vi "LuaVIEW Parse Library Infos.vi"(7 "library path":path, 11 "error in (no error)":errorcluster) -> (8 "library infos":T1[](array[typedef]), 15 "error out":errorcluster)   [LabVIEW 2012]
doc: "Extracts docstrings from a function library and builds a list of function infos."
uses:
  typedefs/clusters/LuaVIEW Function Info.ctl
  served/LuaVIEW Check Synopsis_srv.ctl
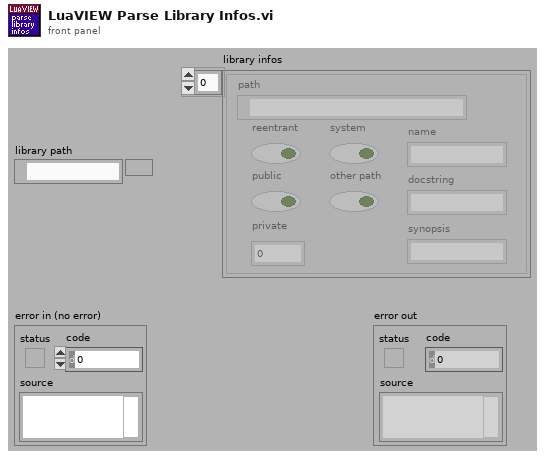
[diagram p1: front panel]
types:
  T1 = typedef "LuaVIEW Function Info.ctl" = cluster{"path":path, "reentrant":bool, "public":bool, "private":i32, "system":bool, "other path":bool, "name":string, "docstring":string, "synopsis":string}
  T2 = typedef "LuaVIEW Check Synopsis_srv.ctl" = refnum<vi>
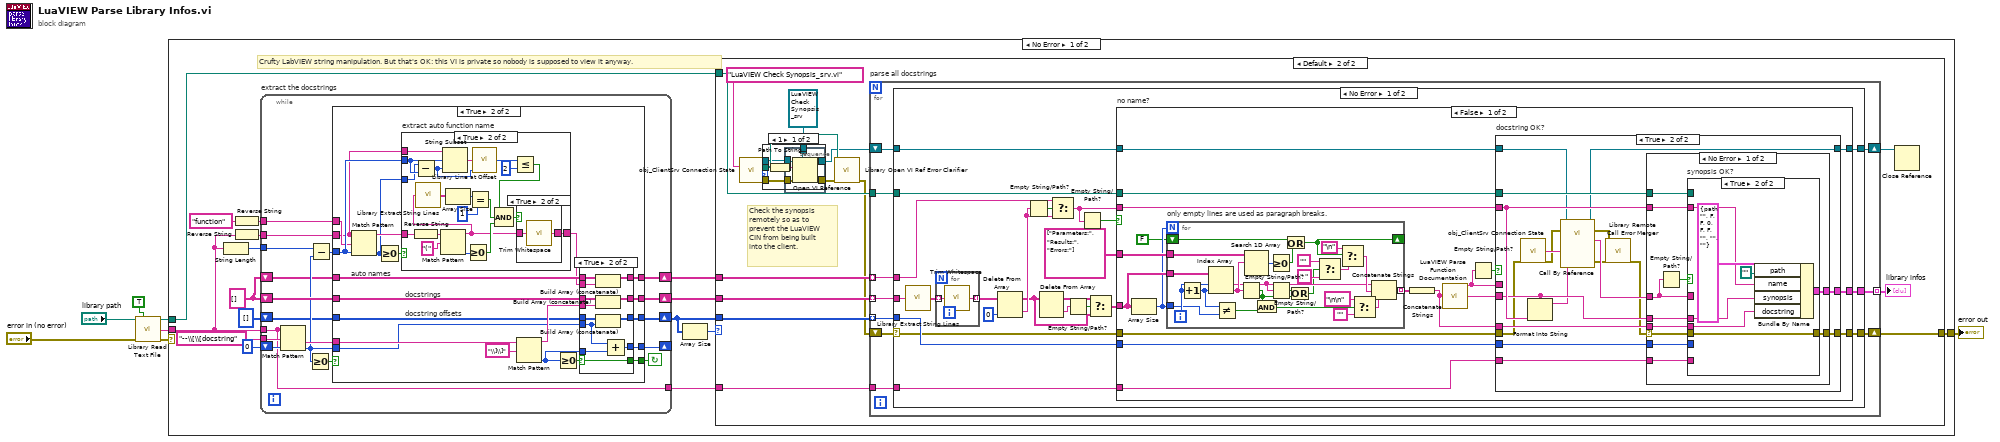
[diagram p0: block diagram]
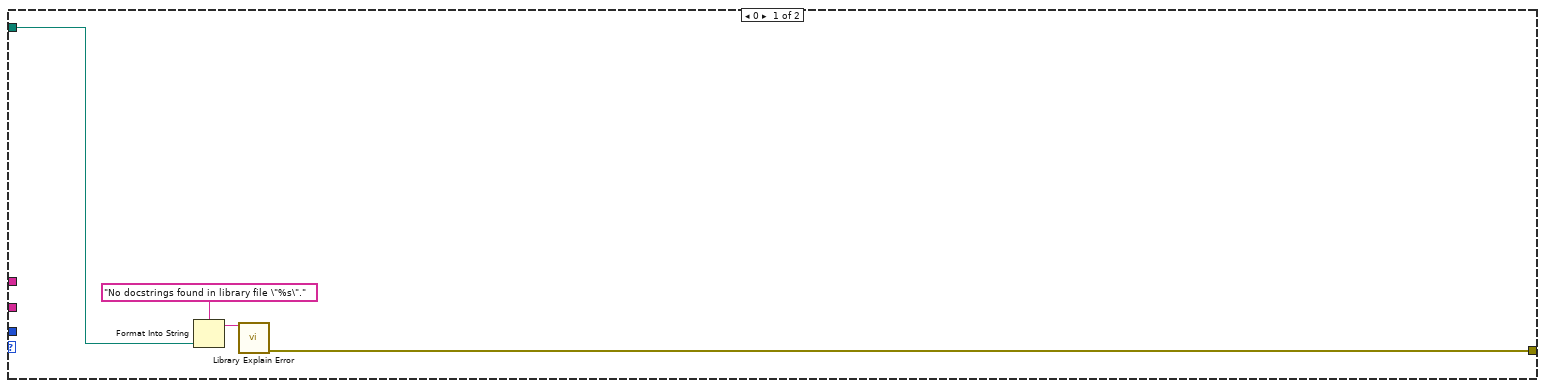
[diagram p2: hidden frame]
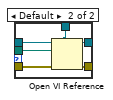
[diagram p3: hidden frame]
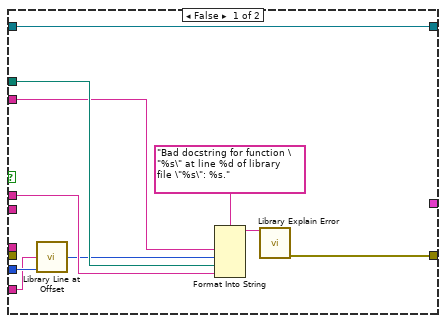
[diagram p4: hidden frame]
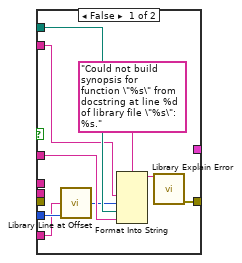
[diagram p5: hidden frame]
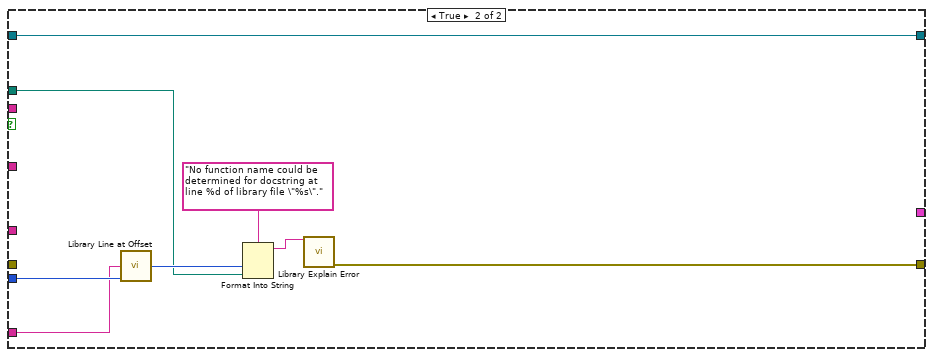
[diagram p7: hidden frame]
diagram:
  n1 = call "Library Read Text File.vi"("file path"="library path", "convert eol (F)"=TRUE, "error in (no error)"="error in (no error)") -> ("dup path"=w1:path, "read text"=w3:string, "error out"=w4:errorcluster)  [unwired: 10 in]
  n2 = case shown="No Error" w4 {
    selector: w4 -> [_ w288]
    tunnel: [w20 w288] -> w7
    tunnel: w3 -> [w18 _]
    tunnel: w1 -> [w19 _]
    frame No Error {
      w12 = string[] []
      # "Crufty LabVIEW string manipulation. But that's OK: this VI is private so nobody is supposed to view it anyway."
      n3 = String Length(string=w18) -> (length=w17:i32)
      n4 = Reverse String(1:"function") -> (0:w13:string)
      n5 = Reverse String(1:w18) -> (0:w14:string)
      n6 = while "extract the docstrings" {
        tunnel: w18 -> [w209]
        shift-right: [w220] -> _
        shift-left: 0 -> [w226]
        shift-right: [w222] -> w22
        shift-left: w12 -> [w223]
        tunnel: w17 -> [w219]
        tunnel: "--\\[\\[docstring" ("regular expression") -> [w216]
        tunnel: w14 -> [w215]
        tunnel: w13 -> [w214]
        shift-right: [w212] -> w11
        shift-left: w12 -> [w213]
        shift-right: [w210] -> w10
        shift-left: i32[] [] -> [w211]
        tunnel: [w209] -> w8
        stop <- w221 continue-if-true
        n7 = Match Pattern(string=w209, regular expression=w216, offset (0)=w226) -> (after substring=w224:string, offset past match=w218:i32)  [unwired: 2 out]
        n8 = Greater Or Equal To 0?(x=w218) -> (x >= 0?=w225:bool)
        n9 = Subtract(x=w219, y=w218) -> (x-y=w217:i32)
        n10 = case shown="True" w225 {
          tunnel: w218 -> [_ w234]
          tunnel: w224 -> [_ w250]
          tunnel: w223 -> [w229 w247]
          tunnel: [w229 w245] -> w222
          tunnel: [_ w244] -> w221
          tunnel: [_ w243] -> w220
          tunnel: w217 -> [_ w233]
          tunnel: w215 -> [_ w230]
          tunnel: w214 -> [_ w231]
          tunnel: w213 -> [w228 w239]
          tunnel: [w228 w237] -> w212
          tunnel: w211 -> [w227 w236]
          tunnel: [w227 w235] -> w210
          frame False {
          }
          frame True {
            # "auto names"
            # "docstrings"
            # "docstring offsets"
            n11 = Match Pattern(string=w230, regular expression=w231, offset (0)=w233) -> (before substring=w240:string, offset past match=w232:i32)  [unwired: 2 out]
            n12 = Greater Or Equal To 0?(x=w232) -> (x >= 0?=w241:bool)
            n13 = case "extract auto function name" shown="True" w241 {
              tunnel: w240 -> [_ w259]
              tunnel: [_ w260] -> w238
              tunnel: w233 -> [_ w258]
              tunnel: w232 -> [_ w257]
              tunnel: w230 -> [_ w256]
              frame False {
              }
              frame True {
                n14 = Subtract(x=w257, y=w258) -> (x-y=w254:i32)
                n15 = Reverse String(1:w259) -> (0:w270:string)
                n16 = Match Pattern(string=w270, regular expression="(") -> (before substring=w265:string, offset past match=w268:i32)  [unwired: 1 in, 2 out]
                n17 = call "Library Extract String Lines.vi"("multi-line string"=w265) -> ("lines"=w264:string[])  [unwired: 14 in]
                n18 = String Subset(string=w256, offset (0)=w258, length (rest)=w254) -> (substring=w255:string)
                n19 = Array Size(array=w264) -> (size(s)=w263:i32)
                n20 = Greater Or Equal To 0?(x=w268) -> (x >= 0?=w267:bool)
                n21 = Equal?(x=w263, y=1) -> (x = y?=w261:bool)
                n22 = call "Library Line at Offset.vi"("multi-line string"=w255, "offset in string"=w254) -> ("line number"=w253:i32)  [unwired: 13 in]
                n23 = Less Or Equal?(x=w253, y=2) -> (x <= y?=w251:bool)
                n24 = Compound Arithmetic op=AND(w251, w261, w267) -> (w266:bool)
                n25 = case shown="True" w266 {
                  tunnel: w265 -> [_ w272]
                  tunnel: [_ w271] -> w260
                  frame False {
                  }
                  frame True {
                    n26 = call <vilib>:"Trim Whitespace.vi"("string"=w272) -> ("trimmed string"=w271:string)  [unwired: 1 in]
                  }
                }
              }
            }
            n27 = Match Pattern(string=w250, regular expression="\\]\\]") -> (before substring=w246:string, offset past match=w242:i32)  [unwired: 1 in, 2 out]
            n28 = Greater Or Equal To 0?(x=w242) -> (x >= 0?=w248:bool)
            n29 = case shown="True" w248 {
              selector: w248 -> [_ w285]
              tunnel: w247 -> [w275 w284]
              tunnel: w246 -> [_ w287]
              tunnel: [w275 w286] -> w245
              tunnel: [_ w285] -> w244
              tunnel: w242 -> [_ w277]
              tunnel: [_ w278] -> w243
              tunnel: w239 -> [w274 w283]
              tunnel: w238 -> [_ w282]
              tunnel: [w274 w281] -> w237
              tunnel: w236 -> [w273 w280]
              tunnel: w234 -> [_ w276]
              tunnel: [w273 w279] -> w235
              frame False {
              }
              frame True {
                n30 = Build Array (concatenate)(w283, w282) -> (w281:string[])
                n31 = Build Array (concatenate)(w284, w287) -> (w286:string[])
                n32 = Build Array (concatenate)(w280, w276) -> (w279:i32[])
                n33 = Add(x=w276, y=w277) -> (x+y=w278:i32)
              }
            }
          }
        }
      }
      n34 = Array Size(array=w10) -> (size(s)=w21:i32)
      n35 = case shown="Default" w21 {
        tunnel: w22 -> [_ w43]
        tunnel: [w26 w40] -> w20
        tunnel: w19 -> [w25 w38]
        tunnel: w11 -> [_ w42]
        tunnel: w10 -> [_ w41]
        tunnel: w8 -> [_ w39]
        frame 0 {
          n36 = Format Into String(format string="No docstrings found in library file \"%s\"." ("explanation"), w25) -> (resulting string=w27:string)  [unwired: 2 in, 1 out]
          n37 = call "Library Explain Error.vi"("explanation prefix (none)"=w27) -> ("explained error"=w26:errorcluster)  [unwired: 14 in]
        }
        frame Default {
          # "Check the synopsis\nremotely so as to\nprevent the LuaVIEW\nCIN from being built\ninto the client."
          n38 = call "obj_ClientSrv Connection State.vi"("machine{connect}/VI{get state} name (local/no path resolution)"="LuaVIEW Check Synopsis_srv.vi") -> ("server app ref"=w30:refnum<vi>, "resolved server path"=w31:path, "error out"=w32:errorcluster)  [unwired: 7 in, 5 out]
          n39 = stacked-sequence {
            tunnel: [w49] -> w28
            tunnel: [w48] -> w33
            tunnel: w32 -> [w47]
            tunnel: w30 -> [w46]
            tunnel: w31 -> [w45]
            tunnel: T2 refnum ("check synopsis") -> [w44]
            frame #0 {
              # "avoid LV8 complaints"
              n40 = Path to Array of Strings(0:w45) -> (2:w50:string[])  [unwired: 1 out]
              n41 = Array Size(array=w50) -> (size(s)=w51:i32)
              n42 = case shown="1" w51 {
                tunnel: w45 -> [w58 w64]
                tunnel: w46 -> [w56 w63]
                tunnel: [w54 w59] -> w49
                tunnel: [w52 w62] -> w48
                tunnel: w44 -> [w53 w61]
                tunnel: w47 -> [w55 w60]
                frame 1 {
                  n43 = Path To String(path=w58) -> (string=w57:string)
                  n44 = Open VI Reference(type specifier VI Refnum (for type only)=w53, application reference (local)=w56, vi path=w57, error in (no error)=w55) -> (vi reference=w54:T2, error out=w52:errorcluster)  [unwired: 2 in]
                }
                frame Default {
                  n45 = Open VI Reference(type specifier VI Refnum (for type only)=w61, application reference (local)=w63, vi path=w64, error in (no error)=w60) -> (vi reference=w59:T2, error out=w62:errorcluster)  [unwired: 2 in]
                }
              }
            }
          }
          n46 = call "Library Open VI Ref Error Clarifier.vi"("VI path"=w31, "called VI error (no error)"=w33) -> ("error out"=w35:errorcluster)  [unwired: 13 in]
          n47 = for "parse all docstrings" {
            tunnel: w43 -> [w74] mode=indexing
            tunnel: w42 -> [w73] mode=indexing
            tunnel: w41 -> [w70] mode=indexing
            shift-right: [w72] -> w40
            shift-left: w35 -> [w71]
            tunnel: w39 -> [w69]
            tunnel: w38 -> [w68]
            tunnel: [w67] -> w37 mode=indexing
            shift-right: [w65] -> w34
            shift-left: w28 -> [w66]
            n48 = case shown="No Error" w71 {
              selector: w71 -> [w84 w208]
              tunnel: w74 -> [w97 _]
              tunnel: w73 -> [w91 _]
              tunnel: [w88 w208] -> w72
              tunnel: w70 -> [w85 _]
              tunnel: w69 -> [w87 _]
              tunnel: w68 -> [w86 _]
              tunnel: [w78 _] -> w67
              tunnel: w66 -> [w77 w207]
              tunnel: [w76 w207] -> w65
              frame No Error {
                n49 = call "Library Extract String Lines.vi"("multi-line string"=w97) -> ("lines"=w96:string[])  [unwired: 14 in]
                n50 = for {
                  tunnel: w96 -> [w206] mode=indexing
                  tunnel: [w205] -> w95 mode=indexing
                  n51 = call <vilib>:"Trim Whitespace.vi"("string"=w206) -> ("trimmed string"=w205:string)  [unwired: 1 in]
                }
                n52 = Delete From Array(array=w95, index=0) -> (deleted portion=w92:string, array with subset deleted=w81:string[])  [unwired: 1 in]
                n53 = Empty String/Path?(string/path=w92) -> (empty?=w93:bool)
                n54 = Delete From Array(array=w81) -> (deleted portion=w83:string, array with subset deleted=w80:string[])  [unwired: 2 in]
                n55 = Select(t=w91, s=w93, f=w92) -> (s? t:f=w89:string)
                n56 = Empty String/Path?(string/path=w83) -> (empty?=w82:bool)
                n57 = Empty String/Path?(string/path=w89) -> (empty?=w90:bool)
                n58 = Select(t=w80, s=w82, f=w81) -> (s? t:f=w79:string[])
                n59 = case "no name?" shown="False" w90 {
                  tunnel: w89 -> [w108 _]
                  tunnel: [w113 w202] -> w88
                  tunnel: w87 -> [w109 w200]
                  tunnel: w86 -> [w105 w198]
                  tunnel: w85 -> [w114 w201]
                  tunnel: w84 -> [w107 _]
                  tunnel: w79 -> [w102 _]
                  tunnel: [w106 _] -> w78
                  tunnel: w77 -> [w104 w197]
                  tunnel: [w103 w197] -> w76
                  tunnel: string[] ["Parameters:", "Results:", "Errors:"] -> [w101 _]
                  frame False {
                    n60 = Array Size(array=w102) -> (size(s)=w99:i32)
                    n61 = for "only empty lines are used as paragraph breaks." {
                      N: w99 -> [_]
                      tunnel: w102 -> [w140]
                      tunnel: w101 -> [w138]
                      tunnel: [w132] -> w100 mode=indexing
                      tunnel: w99 -> [w129]
                      shift-right: [w125] -> _
                      shift-left: FALSE -> [w127]
                      i -> [w139]
                      n62 = Increment(x=w139) -> (x+1=w130:i32)
                      n63 = Index Array(array=w140, index #1=w139, index #2=w130) -> (element #1=w119:string, element #2=w131:string)
                      n64 = Not Equal?(x=w130, y=w129) -> (x != y?=w128:bool)
                      n65 = Empty String/Path?(string/path=w131) -> (empty?=w117:bool)
                      n66 = Search 1D Array(1D array=w138, element=w131) -> (index of element=w137:i32)  [unwired: 1 in]
                      n67 = And(x=w117, y=w128) -> (x .and. y?=w120:bool)
                      n68 = Greater Or Equal To 0?(x=w137) -> (x >= 0?=w126:bool)
                      n69 = Empty String/Path?(string/path=w119) -> (empty?=w118:bool)
                      n70 = Or(x=w127, y=w126) -> (x .or. y?=w125:bool)
                      n71 = Or(x=w118, y=w117) -> (x .or. y?=w116:bool)
                      n72 = Select(t="", s=w116, f=" ") -> (s? t:f=w123:string)
                      n73 = Select(t="\n", s=w125, f=w123) -> (s? t:f=w122:string)
                      n74 = Select(t="\n\n", s=w120, f="") -> (s? t:f=w133:string)
                      n75 = Concatenate Strings(w119, w122, w133) -> (w132:string)
                    }
                    n76 = Concatenate Strings(w100) -> (w110:string)
                    n77 = call "LuaVIEW Parse Function Documentation.vi"("documentation"=w110) -> ("formatting error"=w112:string, "unnamed synopsis"=w111:string)  [unwired: 13 in]
                    n78 = Empty String/Path?(string/path=w112) -> (empty?=w115:bool)
                    n79 = case "docstring OK?" shown="True" w115 {
                      tunnel: w105 -> [w148 w168]
                      tunnel: w114 -> [w147 w166]
                      tunnel: [w146 w167] -> w113
                      tunnel: w112 -> [w145 _]
                      tunnel: w111 -> [_ w162]
                      tunnel: w110 -> [_ w164]
                      tunnel: w109 -> [w144 w165]
                      tunnel: w108 -> [w142 w163]
                      tunnel: w107 -> [_ w152]
                      tunnel: [_ w161] -> w106
                      tunnel: w104 -> [w141 w151]
                      tunnel: [w141 w153] -> w103
                      frame False {
                        n80 = call "Library Line at Offset.vi"("multi-line string"=w144, "offset in string"=w147) -> ("line number"=w143:i32)  [unwired: 13 in]
                        n81 = Format Into String(format string="Bad docstring for function \"%s\" at line %d of library file \"%s\": %s." ("explanation"), w142, w143, w148, w145) -> (resulting string=w150:string)  [unwired: 2 in, 1 out]
                        n82 = call "Library Explain Error.vi"("explanation prefix (none)"=w150) -> ("explained error"=w146:errorcluster)  [unwired: 14 in]
                      }
                      frame True {
                        n83 = call "obj_ClientSrv Connection State.vi"("error in (no error)"=w152) -> ("observer certificate"=w160:string, "error out"=w159:errorcluster)  [unwired: 7 in, 6 out]
                        n84 = Format Into String(format string=w162, w163) -> (resulting string=w158:string)  [unwired: 2 in, 1 out]
                        n85 = call-by-ref "?"(reference=w151, error in=w159, "certificate"=w160, "synopsis"=w158) -> (reference out=w153:T2, error out=w154:errorcluster, "synopsis error"=w157:string, 15:"error out"=w155:errorcluster)  [unwired: 12 in]
                        n86 = call "Library Remote Call Error Merger.vi"("call by reference node error"=w154, "called VI error (no error)"=w155) -> ("error out"=w156:errorcluster)  [unwired: 13 in]
                        n87 = case shown="No Error" w156 {
                          selector: w156 -> [w169 w196]
                          tunnel: w168 -> [w178 _]
                          tunnel: [w177 w196] -> w167
                          tunnel: w166 -> [w176 _]
                          tunnel: w165 -> [w175 _]
                          tunnel: w164 -> [w174 _]
                          tunnel: w163 -> [w173 _]
                          tunnel: w162 -> [w172 _]
                          tunnel: [w171 _] -> w161
                          tunnel: w157 -> [w170 _]
                          frame No Error {
                            n88 = Empty String/Path?(string/path=w170) -> (empty?=w179:bool)
                            n89 = case "synopsis OK?" shown="True" w179 {
                              tunnel: w170 -> [w185 _]
                              tunnel: w178 -> [w186 _]
                              tunnel: [w184 w191] -> w177
                              tunnel: w176 -> [w183 _]
                              tunnel: w175 -> [w182 _]
                              tunnel: w174 -> [_ w192]
                              tunnel: w173 -> [w180 w194]
                              tunnel: w172 -> [_ w193]
                              tunnel: w169 -> [_ w191]
                              tunnel: [_ w190] -> w171
                              frame False {
                                n90 = call "Library Line at Offset.vi"("multi-line string"=w182, "offset in string"=w183) -> ("line number"=w181:i32)  [unwired: 13 in]
                                n91 = Format Into String(format string="Could not build synopsis for function \"%s\" from docstring at line %d of library file \"%s\": %s." ("explanation"), w180, w181, w186, w185) -> (resulting string=w188:string)  [unwired: 2 in, 1 out]
                                n92 = call "Library Explain Error.vi"("explanation prefix (none)"=w188) -> ("explained error"=w184:errorcluster)  [unwired: 14 in]
                              }
                              frame True {
                                n93 = Bundle By Name(cluster=T1 {"path"=path "", "reentrant"=FALSE, "public"=FALSE, "private"=0, "system"=FALSE, "other path"=FALSE, "name"="", "docstring"="", "synopsis"=""} ("function info"), "path"=path "", "name"=w194, "synopsis"=w193, "docstring"=w192) -> (w190:T1)
                              }
                            }
                          }
                          frame Error {
                          }
                        }
                      }
                    }
                  }
                  frame True {
                    n94 = call "Library Line at Offset.vi"("multi-line string"=w200, "offset in string"=w201) -> ("line number"=w199:i32)  [unwired: 13 in]
                    n95 = Format Into String(format string="No function name could be determined for docstring at line %d of library file \"%s\"." ("explanation"), w199, w198) -> (resulting string=w204:string)  [unwired: 2 in, 1 out]
                    n96 = call "Library Explain Error.vi"("explanation prefix (none)"=w204) -> ("explained error"=w202:errorcluster)  [unwired: 14 in]
                  }
                }
              }
              frame Error {
              }
            }
          }
          "library infos" <- w37
          n97 = Close Reference(reference=w34) -> ()  [unwired: 1 in, 1 out]
        }
      }
    }
    frame Error {
    }
  }
  "error out" <- w7
